vi "arm_kinematics (SubVI).vi"(3 "alpha":dbl, 4 "y":dbl, 5 "x":dbl) -> (0 "R":dbl, 1 "alpha":dbl, 2 "teta":dbl)   [LabVIEW 2017]
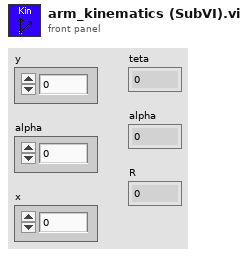
[diagram p1: front panel]
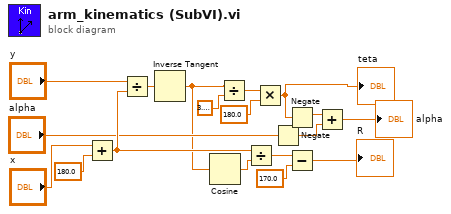
[diagram p0: block diagram]
diagram:
  n1 = Add(x="x", y=180.0) -> (x+y=w12:dbl)
  n2 = Divide(x="y", y=w12) -> (x/y=w8:dbl)
  n3 = Inverse Tangent(1:w8) -> (0:w5:dbl)
  n4 = Cosine(x=w5) -> (cos(x)=w16:dbl)
  n5 = Divide(x=w5, y=3.141592653589793) -> (x/y=w3:dbl)
  n6 = Divide(x=w12, y=w16) -> (x/y=w13:dbl)
  n7 = Multiply(x=w3, y=180.0) -> (x*y=w2:dbl)
  "teta" <- w2
  n8 = Negate(x="alpha") -> (-x=w6:dbl)
  n9 = Negate(x=w2) -> (-x=w18:dbl)
  n10 = Subtract(x=w13, y=170.0) -> (x-y=→"R":dbl)
  n11 = Add(x=w18, y=w6) -> (x+y=→"alpha":dbl)
